vi "EventInfoCustomEvent.vi"(3 "eventstr":string) -> (0 "error out":errorcluster, 1 "JSON Tree out (JSON Object)":variant)   [LabVIEW 2018]
uses:
  <vilib>/LVH/i3 JSON/JSON Generation/Create Value Files/Create Value - Object.vi
  <vilib>/LVH/i3 JSON/JSON Generation/Add Object Parameter Files/Add Object Parameter - String.vi
  <vilib>/LVH/i3 JSON/JSON Generation/Add Object Parameter Files/Add Object Parameter - Object.vi
  <vilib>/LVH/i3 JSON/i3-json.lvlib
panel:
  in  "error in (no error)":errorcluster
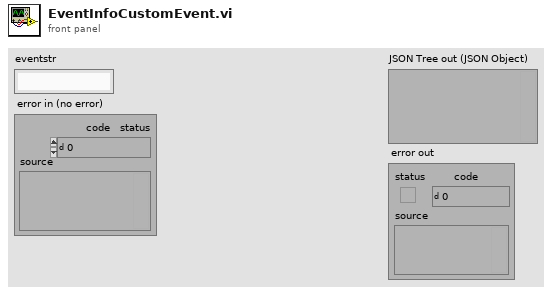
[diagram p1: front panel]
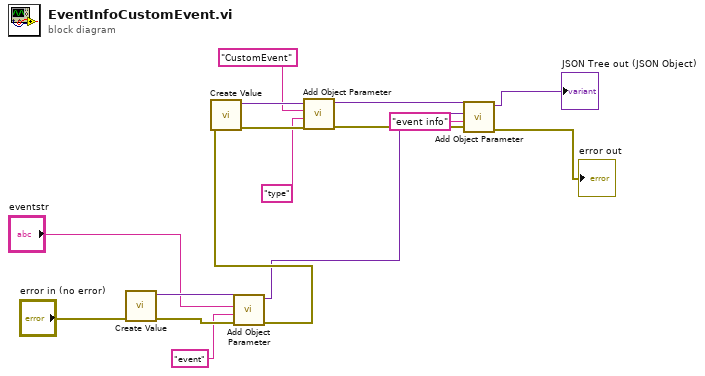
[diagram p0: block diagram]
diagram:
  n1 = call-poly <vilib>:"Create Value.vi"("error in (no error)"="error in (no error)") -> ("error out"=w15:errorcluster, "JSON Tree"=w16:variant)  [unwired: 9 in]
  n2 = call-poly <vilib>:"Add Object Parameter.vi"("error in (no error)"=w15, "Name"="event", "String"="eventstr", "JSON Tree in (JSON Object)"=w16) -> ("error out"=w5:errorcluster, "JSON Tree out (JSON Object)"=w4:variant)  [unwired: 6 in]
  n3 = call-poly <vilib>:"Create Value.vi"("error in (no error)"=w5) -> ("error out"=w10:errorcluster, "JSON Tree"=w11:variant)  [unwired: 9 in]
  n4 = call-poly <vilib>:"Add Object Parameter.vi"("error in (no error)"=w10, "Name"="type", "String"="CustomEvent", "JSON Tree in (JSON Object)"=w11) -> ("error out"=w7:errorcluster, "JSON Tree out (JSON Object)"=w6:variant)  [unwired: 6 in]
  n5 = call-poly <vilib>:"Add Object Parameter.vi"("error in (no error)"=w7, "Name"="event info", "JSON Object"=w4, "JSON Tree in (JSON Object)"=w6) -> ("error out"=→"error out":errorcluster, "JSON Tree out (JSON Object)"=→"JSON Tree out (JSON Object)":variant)  [unwired: 6 in]
